vi "Constructor.vi"(8 "error in (no error)":errorcluster, 9 "FPGA Template Path":path, 10 "FPGA Target Name":string, 11 "Project Path":path) -> (0 "error out":errorcluster, 3 "Project out":refnum<class "Project.lvclass">)   [LabVIEW 2015, in "Project.lvclass"]
uses:
  Project.lvclass
  Project.lvclass/Project.ctl
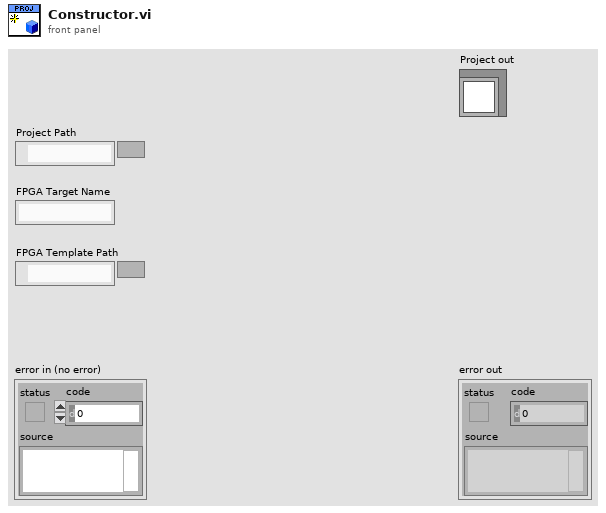
[diagram p1: front panel]
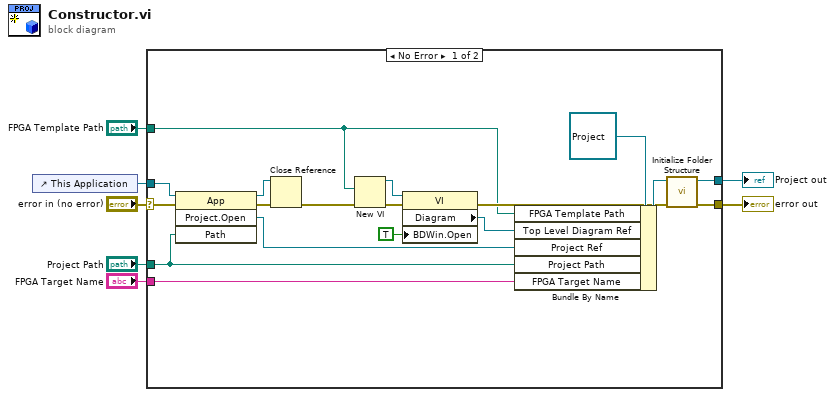
[diagram p0: block diagram]
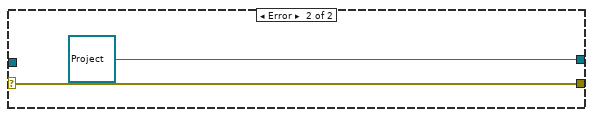
[diagram p2: hidden frame]
diagram:
  n1 = control-ref of="This Application"() -> (w1:refnum<vi>)
  n2 = case shown="No Error" "error in (no error)" {
    selector: "error in (no error)" -> [w22 w27]
    tunnel: [w21 w27] -> w6
    tunnel: [w19 refnum<class "Project.lvclass"> refnum ("Project out")] -> w5
    tunnel: "Project Path" -> [w12 _]
    tunnel: "FPGA Target Name" -> [w11 _]
    tunnel: "FPGA Template Path" -> [w9 _]
    tunnel: w1 -> [w8 _]
    frame No Error {
      n3 = invoke class="App" method="Project.Open"(reference=w8, error in=w22, "Path"=w12) -> (reference out=w24:refnum<vi>, error out=w25:errorcluster, "Project:Open"=w23:refnum<vi>)  [unwired: 1 in, 1 out]
      n4 = Close Reference(reference=w24, error in (no error)=w25) -> (error out=w14:errorcluster)
      n5 = New VI(8:w14, 10:w9) -> (0:w16:errorcluster, 3:w17:refnum<vi>)  [unwired: 5 in]
      n6 = property class="VI"(reference=w17, error in=w16, "BDWin.Open"=TRUE ("Block Diagram Window:Open")) -> (error out=w13:errorcluster, "Diagram"=w10:refnum<vi>)  [unwired: 1 out]
      n7 = Bundle By Name(cluster=refnum<class "Project.lvclass"> refnum ("Project out"), "FPGA Template Path"=w9, "Top Level Diagram Ref"=w10, "Project Ref"=w23, "Project Path"=w12, "FPGA Target Name"=w11) -> (w20:refnum<class "Project.lvclass">)
      n8 = call-dynamic "Initialize Folder Structure.vi"("error in (no error)"=w13, "Project in"=w20) -> ("error out"=w21:errorcluster, "Project out"=w19:refnum<class "Project.lvclass">)  [unwired: 8 in]
    }
    frame Error {
    }
  }
  "error out" <- w6
  "Project out" <- w5
